vi "Write 2D Double.vi"(10 "2D Double":dbl[][](array[numeric]), 11 "_Message (2D Double) in":refnum<class "_Message (2D Double).lvclass">) -> (3 "_Message (2D Double) out":refnum<class "_Message (2D Double).lvclass">)   [LabVIEW 2016, in "MVC Subscription.lvlib" / "_Message (2D Double).lvclass"]
uses:
  _Message (2D Double).lvclass
  _Message (2D Double).lvclass/_Message (2D Double).ctl
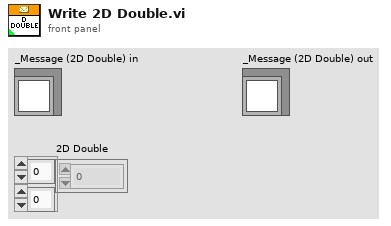
[diagram p1: front panel]
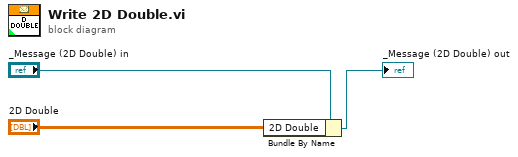
[diagram p0: block diagram]
diagram:
  n1 = Bundle By Name(cluster="_Message (2D Double) in", "2D Double"="2D Double") -> (→"_Message (2D Double) out":refnum<class "_Message (2D Double).lvclass">)
